vi "Main.vi"(8 "error in":errorcluster, 11 "Fluke DMM in":refnum<class "Fluke DMM.lvclass">) -> (0 "error out":errorcluster, 3 "Fluke DMM out":refnum<class "Fluke DMM.lvclass">)   [LabVIEW 2020, in "Fluke DMM.lvclass"]
doc: "The <b>Queued Message Handler</b> of the Worker that owns this VI."
uses:
  Fluke DMM.lvclass
  Initialization Data.ctl
  Response Cases.ctl
  Fluke DMM.lvclass/Fluke DMM.ctl
  Interfaces/DMM HAL/rwr_Set Measurement Type.ctl
  Interfaces/DMM HAL/rwr_Set Measurement Type Reply.ctl
  Interfaces/DMM HAL/rwr_Set Voltage Range.ctl
  Interfaces/DMM HAL/rwr_Set Voltage Range Reply.ctl
  Interfaces/DMM HAL/rwr_Start Measurement.ctl
  Interfaces/DMM HAL/rwr_Start Measurement Reply.ctl
  Interfaces/DMM HAL/rwr_Stop Measurement.ctl
  Interfaces/DMM HAL/rwr_Stop Measurement Reply.ctl
  Interfaces/DMM HAL/rwr_Read Measurement.ctl
  Interfaces/DMM HAL/rwr_Read Measurement Reply.ctl
  Interfaces/DMM HAL/rqp_Set Current Range.ctl
  <vilib>/Utility/error.llb/Error Cluster From Error Code.vi
  <vilib>/ErrorRing/Error Ring.xnode
  Interfaces/DMM HAL/DMM HAL.lvclass
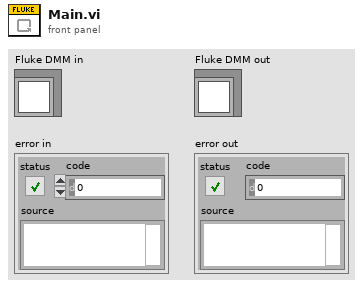
[diagram p1: front panel]
types:
  T1 = typedef "Fluke DMM.lvclass/Initialization Data.ctl" = cluster{"Response Cases":T2}
  T2 = typedef "Fluke DMM.lvclass/Response Cases.ctl" = cluster{"Placeholder - Can be deleted":string}
  T3 = typedef "DMM HAL.lvclass/rwr_Set Measurement Type Reply.ctl" = cluster{"String":string}
  T4 = typedef "DMM HAL.lvclass/rwr_Set Measurement Type.ctl" = cluster{"String":string}
  T5 = typedef "DMM HAL.lvclass/rwr_Set Voltage Range Reply.ctl" = cluster{"String":string}
  T6 = typedef "DMM HAL.lvclass/rwr_Set Voltage Range.ctl" = cluster{"String":string}
  T7 = typedef "DMM HAL.lvclass/rwr_Start Measurement Reply.ctl" = cluster{"String":string}
  T8 = typedef "DMM HAL.lvclass/rwr_Start Measurement.ctl" = cluster{"String":string}
  T9 = typedef "DMM HAL.lvclass/rwr_Stop Measurement Reply.ctl" = cluster{"String":string}
  T10 = typedef "DMM HAL.lvclass/rwr_Stop Measurement.ctl" = cluster{"String":string}
  T11 = typedef "DMM HAL.lvclass/rwr_Read Measurement Reply.ctl" = cluster{"Numeric":dbl}
  T12 = typedef "DMM HAL.lvclass/rwr_Read Measurement.ctl" = cluster{"String":string}
  T13 = typedef "DMM HAL.lvclass/rqp_Set Current Range.ctl" = cluster{"String":string}
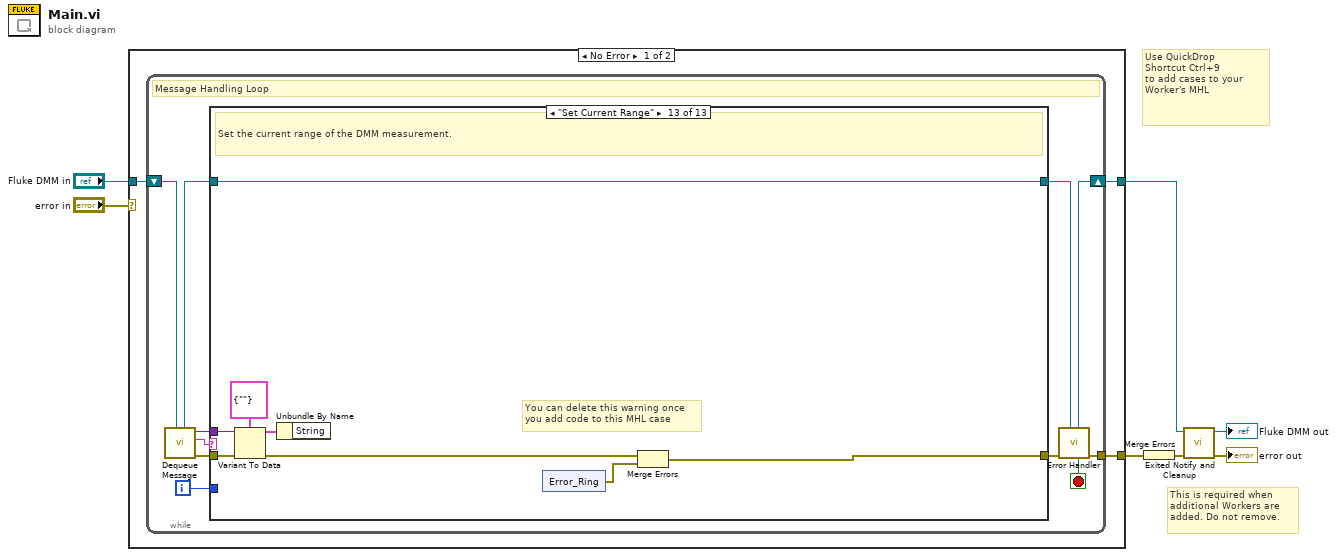
[diagram p0: block diagram]
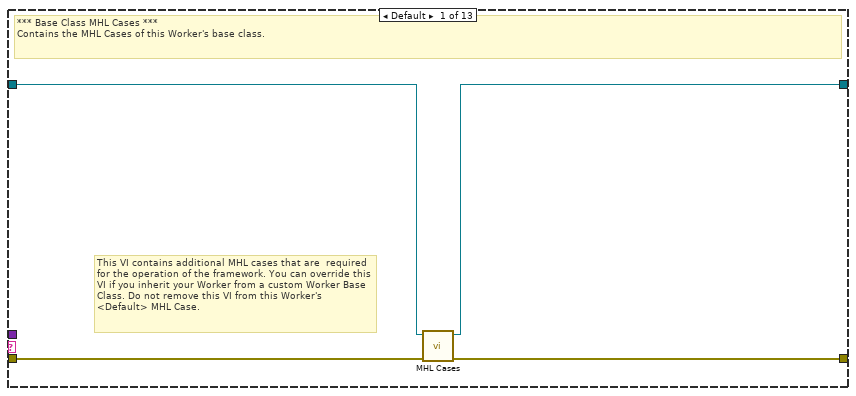
[diagram p2: hidden frame]
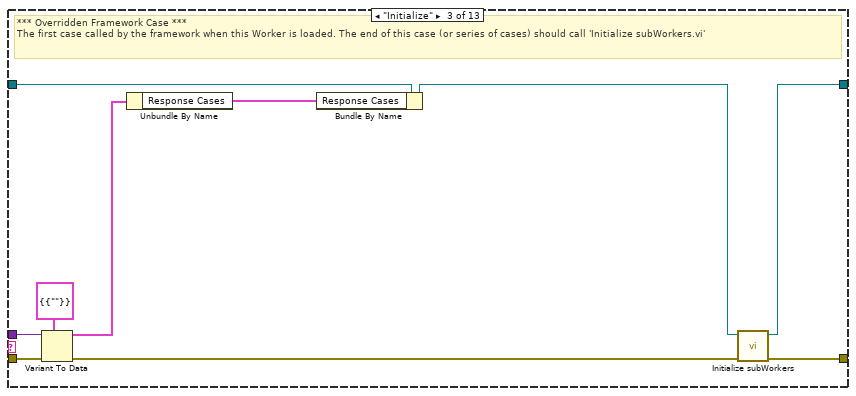
[diagram p4: hidden frame]
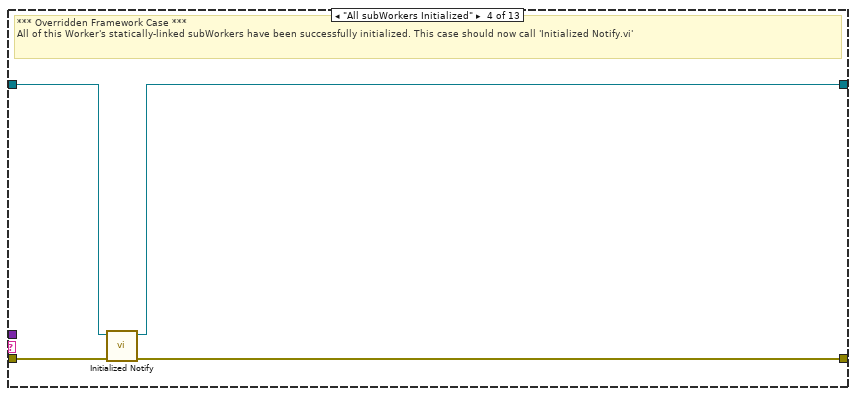
[diagram p5: hidden frame]
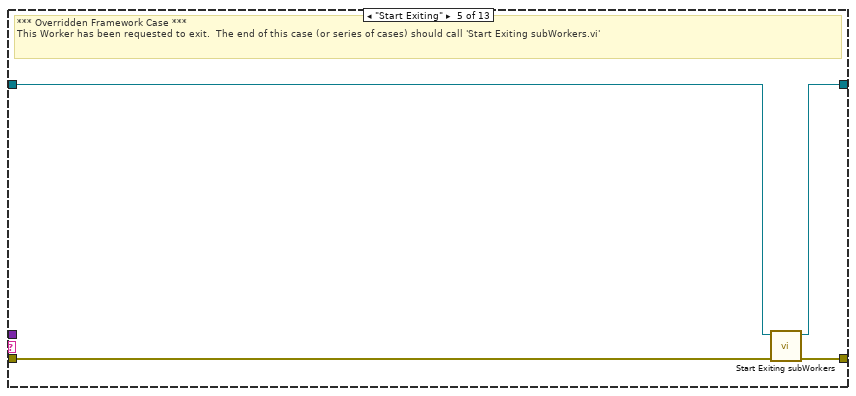
[diagram p6: hidden frame]
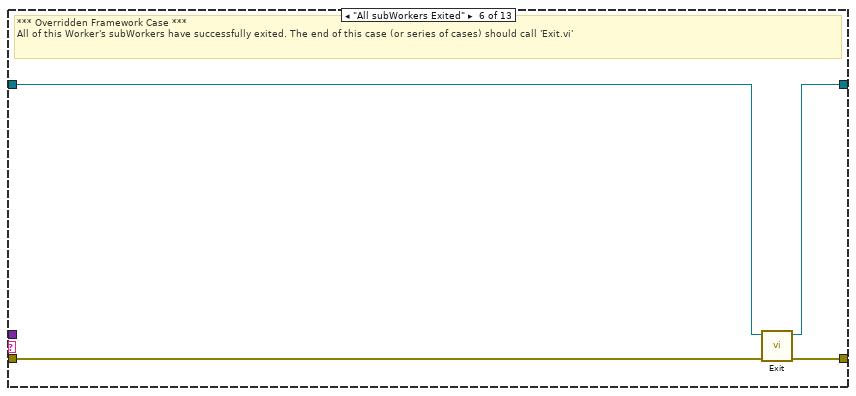
[diagram p7: hidden frame]
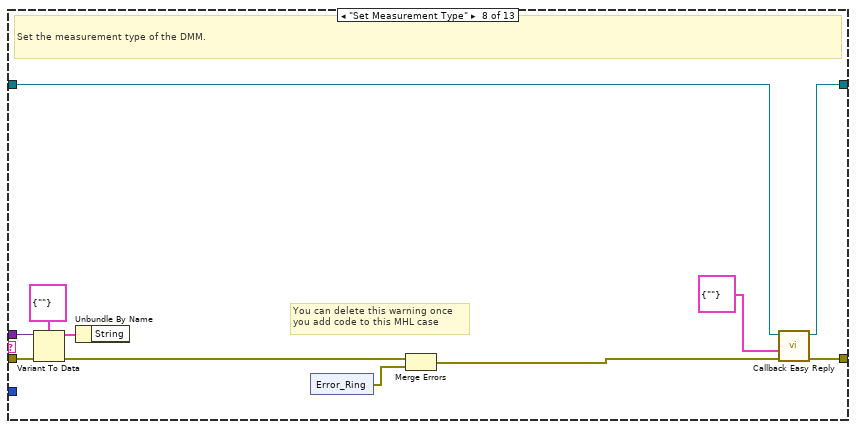
[diagram p9: hidden frame]
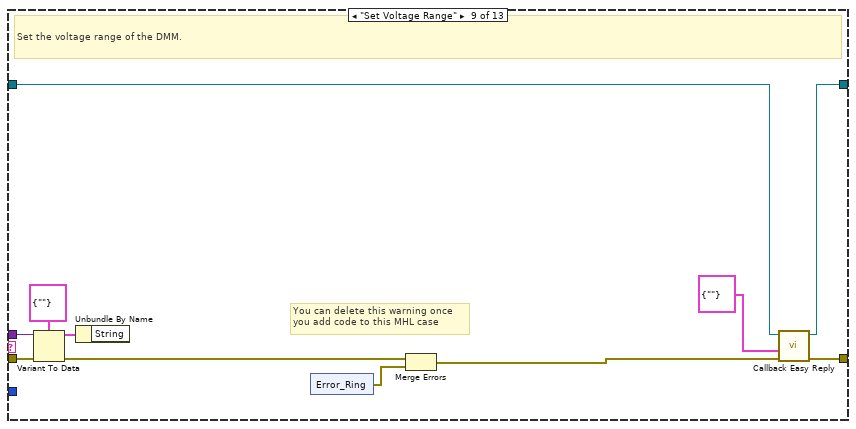
[diagram p10: hidden frame]
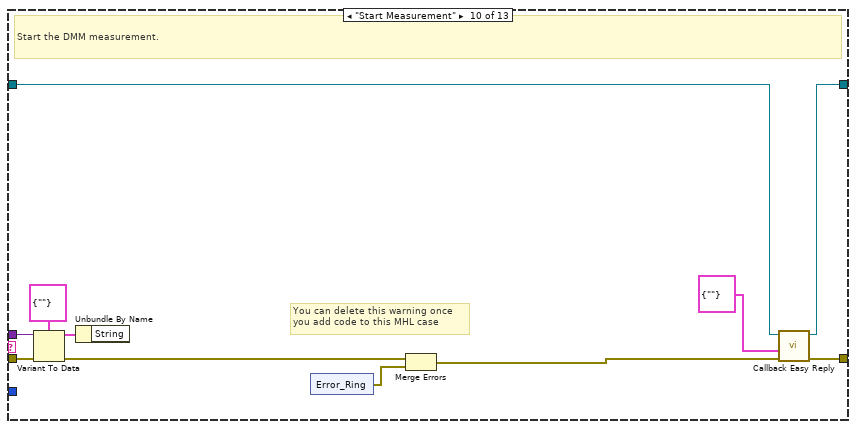
[diagram p11: hidden frame]
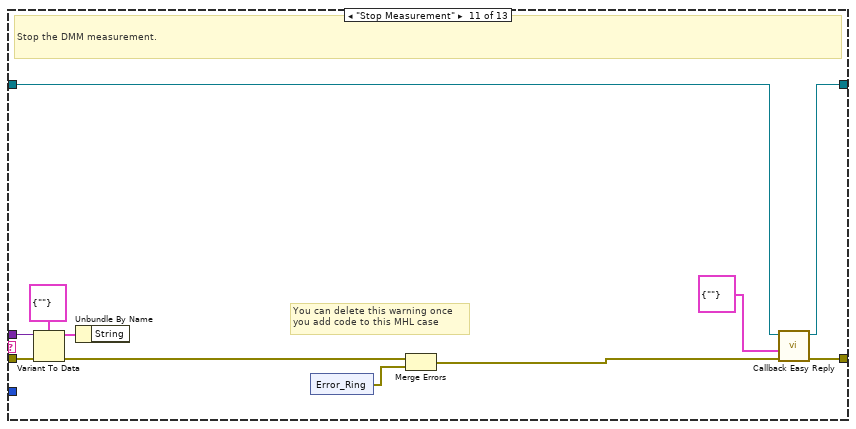
[diagram p12: hidden frame]
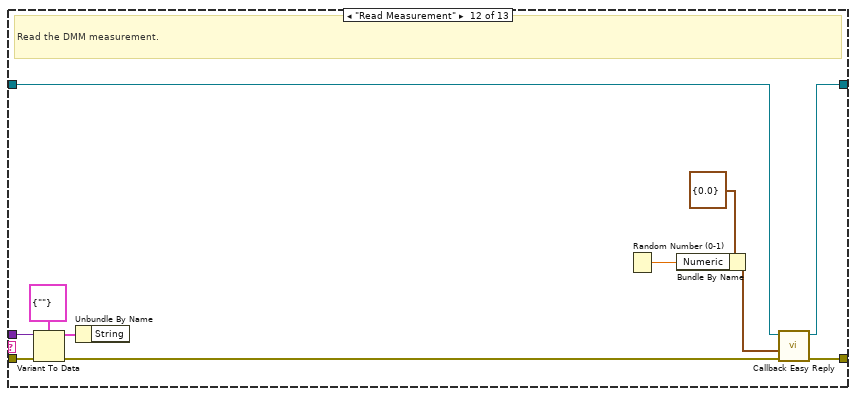
[diagram p13: hidden frame]
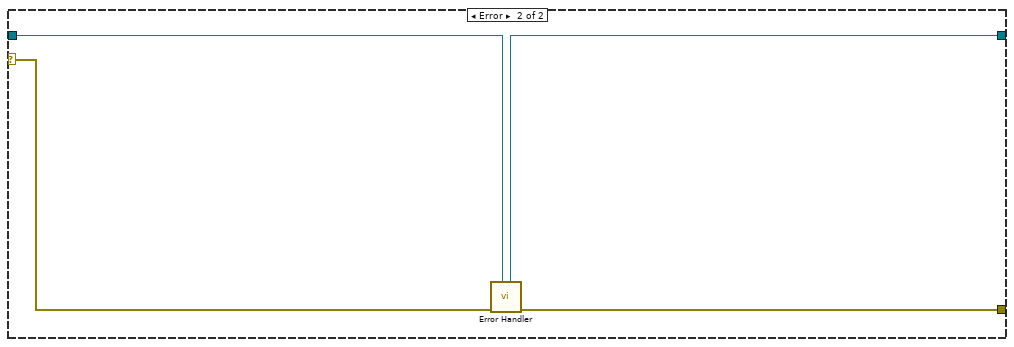
[diagram p14: hidden frame]
diagram:
  # "Use QuickDrop\nShortcut Ctrl+9\nto add cases to your\nWorker's MHL"
  # "This is required when additional Workers are added. Do not remove."
  n1 = case shown="No Error" "error in" {
    tunnel: "Fluke DMM in" -> [w8 w141]
    tunnel: [w10 w142] -> w6
    tunnel: [w9 w140] -> w7
    selector: "error in" -> [_ w143]
    frame No Error {
      n2 = while {
        shift-right: [w19] -> w9
        shift-left: w8 -> [w21]
        tunnel: [w20] -> w10
        i -> [w12]
        stop <- w13 stop-if-true
        # "Message Handling Loop"
        n3 = call-dynamic "Dequeue Message.vi"("Worker"=w21) -> ("error out"=w18:errorcluster, "Case out"=w14:string, "Data out"=w11:variant, "Worker out"=w16:refnum<class "Fluke DMM.lvclass">)  [unwired: 6 in, 1 out]
        n4 = case "Worker MHL Case Structure (DO NOT CHANGE LABEL NAME)" shown="\"Set Current Range\"" w14 {
          tunnel: w18 -> [w25 w26 w35 w41 w42 w49 w51 w62 w78 w94 w110 w126 w133]
          tunnel: [w24 w26 w37 w40 w45 w48 w51 w57 w73 w89 w105 w121 w128] -> w17
          tunnel: w16 -> [w23 w27 w34 w39 w43 w47 w50 w55 w71 w87 w103 w119 w134]
          tunnel: [w22 w27 w36 w38 w44 w46 w50 w56 w72 w88 w104 w120 w134] -> w15
          tunnel: w12 -> [_ _ _ _ _ _ _ _ _ _ _ _ _]
          tunnel: w11 -> [_ _ w32 _ _ _ _ w59 w75 w91 w107 w123 w130]
          frame Default {
            # "This VI contains additional MHL cases that are  required for the operation of the framework. You can override this VI if you inherit your Worker from a custom Worker Base Class. Do not remove this VI from this Worker's <Default> MHL Case."
            # "*** Base Class MHL Cases ***\nContains the MHL Cases of this Worker's base class."
            n5 = call-dynamic "MHL Cases.vi"("error in"=w25, "Worker in"=w23) -> ("error out"=w24:errorcluster, "Worker out"=w22:refnum<class "Fluke DMM.lvclass">)  [unwired: 8 in]
          }
          frame "------------ FRAMEWORK CASES -----------" {
            # "Start of Workers Framework Cases"
          }
          frame "Initialize" {
            # "*** Overridden Framework Case ***\nThe first case called by the framework when this Worker is loaded. The end of this case (or series of cases) should call 'Initialize subWorkers.vi'"
            n6 = Variant To Data(error in=w35, type=T1 {"Response Cases"={"Placeholder - Can be deleted"=""}} ("Cluster"), Variant=w32) -> (data=w30:T1, error out=w33:errorcluster)
            n7 = Unbundle By Name(w30) -> ("Response Cases"=w29:T2)
            n8 = Bundle By Name(cluster=w34, "Response Cases"=w29) -> (w31:refnum<class "Fluke DMM.lvclass">)
            n9 = call-dynamic "Initialize subWorkers.vi"("error in"=w33, "Worker"=w31) -> ("error out"=w37:errorcluster, "dup Worker out"=w36:refnum<class "Fluke DMM.lvclass">)  [unwired: 8 in]
          }
          frame "All subWorkers Initialized" {
            # "*** Overridden Framework Case ***\nAll of this Worker's statically-linked subWorkers have been successfully initialized. This case should now call 'Initialized Notify.vi'"
            n10 = call-dynamic "Initialized Notify.vi"("error in"=w41, "Worker"=w39) -> ("error out"=w40:errorcluster, "dup Worker out"=w38:refnum<class "Fluke DMM.lvclass">)  [unwired: 8 in]
          }
          frame "Start Exiting" {
            # "*** Overridden Framework Case ***\nThis Worker has been requested to exit.  The end of this case (or series of cases) should call 'Start Exiting subWorkers.vi'"
            n11 = call-dynamic "Start Exiting subWorkers.vi"("error_in"=w42, "Worker"=w43) -> ("error out"=w45:errorcluster, "dup Worker out"=w44:refnum<class "Fluke DMM.lvclass">)  [unwired: 8 in]
          }
          frame "All subWorkers Exited" {
            # "*** Overridden Framework Case ***\nAll of this Worker's subWorkers have successfully exited. The end of this case (or series of cases) should call 'Exit.vi'"
            n12 = call-dynamic "Exit.vi"("error_in"=w49, "Worker"=w47) -> ("error out"=w48:errorcluster, "dup Worker out"=w46:refnum<class "Fluke DMM.lvclass">)  [unwired: 8 in]
          }
          frame "------------- PUBLIC API CASES -------------" {
            # "Start of Workers Public API Cases"
          }
          frame "Set Measurement Type" {
            # "You can delete this warning once\nyou add code to this MHL case"
            # "Set the measurement type of the DMM."
            n13 = Variant To Data(error in=w62, type=T4 {"String"=""} ("Data"), Variant=w59) -> (data=w58:T4, error out=w61:errorcluster)
            n14 = Unbundle By Name(w58) -> ()  [unwired: 1 out]
            n15 = xnode ("Error_Ring")() -> ("error out"=w52:errorcluster)
            n16 = Merge Errors(w61, w52) -> (w53:errorcluster)
            n17 = call-dynamic "Callback Easy Reply.vi"("error in"=w53, "Data"=T3 {"String"=""} ("Reply Data"), "Worker"=w55) -> ("error out"=w57:errorcluster, "dup Worker out"=w56:refnum<class "Fluke DMM.lvclass">)  [unwired: 7 in]
          }
          frame "Set Voltage Range" {
            # "You can delete this warning once\nyou add code to this MHL case"
            # "Set the voltage range of the DMM."
            n18 = Variant To Data(error in=w78, type=T6 {"String"=""} ("Data"), Variant=w75) -> (data=w74:T6, error out=w77:errorcluster)
            n19 = Unbundle By Name(w74) -> ()  [unwired: 1 out]
            n20 = xnode ("Error_Ring")() -> ("error out"=w68:errorcluster)
            n21 = Merge Errors(w77, w68) -> (w69:errorcluster)
            n22 = call-dynamic "Callback Easy Reply.vi"("error in"=w69, "Data"=T5 {"String"=""} ("Reply Data"), "Worker"=w71) -> ("error out"=w73:errorcluster, "dup Worker out"=w72:refnum<class "Fluke DMM.lvclass">)  [unwired: 7 in]
          }
          frame "Start Measurement" {
            # "You can delete this warning once\nyou add code to this MHL case"
            # "Start the DMM measurement."
            n23 = Variant To Data(error in=w94, type=T8 {"String"=""} ("Data"), Variant=w91) -> (data=w90:T8, error out=w93:errorcluster)
            n24 = Unbundle By Name(w90) -> ()  [unwired: 1 out]
            n25 = xnode ("Error_Ring")() -> ("error out"=w84:errorcluster)
            n26 = Merge Errors(w93, w84) -> (w85:errorcluster)
            n27 = call-dynamic "Callback Easy Reply.vi"("error in"=w85, "Data"=T7 {"String"=""} ("Reply Data"), "Worker"=w87) -> ("error out"=w89:errorcluster, "dup Worker out"=w88:refnum<class "Fluke DMM.lvclass">)  [unwired: 7 in]
          }
          frame "Stop Measurement" {
            # "You can delete this warning once\nyou add code to this MHL case"
            # "Stop the DMM measurement."
            n28 = Variant To Data(error in=w110, type=T10 {"String"=""} ("Data"), Variant=w107) -> (data=w106:T10, error out=w109:errorcluster)
            n29 = Unbundle By Name(w106) -> ()  [unwired: 1 out]
            n30 = xnode ("Error_Ring")() -> ("error out"=w100:errorcluster)
            n31 = Merge Errors(w109, w100) -> (w101:errorcluster)
            n32 = call-dynamic "Callback Easy Reply.vi"("error in"=w101, "Data"=T9 {"String"=""} ("Reply Data"), "Worker"=w103) -> ("error out"=w105:errorcluster, "dup Worker out"=w104:refnum<class "Fluke DMM.lvclass">)  [unwired: 7 in]
          }
          frame "Read Measurement" {
            # "Read the DMM measurement."
            n33 = Variant To Data(error in=w126, type=T12 {"String"=""} ("Data"), Variant=w123) -> (data=w122:T12, error out=w125:errorcluster)
            n34 = Unbundle By Name(w122) -> ()  [unwired: 1 out]
            n35 = Random Number (0-1)() -> (number: 0 to 1=w116:dbl)
            n36 = Bundle By Name(cluster=T11 {"Numeric"=0.0} ("Reply Data"), "Numeric"=w116) -> (w117:T11)
            n37 = call-dynamic "Callback Easy Reply.vi"("error in"=w125, "Data"=w117, "Worker"=w119) -> ("error out"=w121:errorcluster, "dup Worker out"=w120:refnum<class "Fluke DMM.lvclass">)  [unwired: 7 in]
          }
          frame "Set Current Range" {
            # "You can delete this warning once\nyou add code to this MHL case"
            # "Set the current range of the DMM measurement."
            n38 = Variant To Data(error in=w133, type=T13 {"String"=""} ("Data"), Variant=w130) -> (data=w129:T13, error out=w132:errorcluster)
            n39 = Unbundle By Name(w129) -> ()  [unwired: 1 out]
            n40 = xnode ("Error_Ring")() -> ("error out"=w127:errorcluster)
            n41 = Merge Errors(w132, w127) -> (w128:errorcluster)
          }
        }
        n42 = call-dynamic "Error Handler.vi"("Worker"=w15, "error_in"=w17) -> ("error out"=w20:errorcluster, "Stop Loop"=w13:bool, "Worker out"=w19:refnum<class "Fluke DMM.lvclass">)  [unwired: 7 in]
      }
    }
    frame Error {
      n43 = call-dynamic "Error Handler.vi"("Worker"=w141, "error_in"=w143) -> ("error out"=w142:errorcluster, "Worker out"=w140:refnum<class "Fluke DMM.lvclass">)  [unwired: 7 in, 1 out]
    }
  }
  n44 = Merge Errors(w6) -> (w3:errorcluster)
  n45 = call-dynamic "Exited Notify and Cleanup.vi"("error_in"=w3, "Worker"=w7) -> ("error out"=→"error out":errorcluster, "dup Worker out"=→"Fluke DMM out":refnum<class "Fluke DMM.lvclass">)  [unwired: 8 in]
